vi "UnloadAction.vi"(8 "error in (no error)":errorcluster caption="entrée d'erreur (pas d'erreur)", 11 "Tools In":refnum<class "LeafMagnetometer.lvclass"> caption="DNL_LabVIEW Object in") -> (0 "error out":errorcluster caption="sortie d'erreur", 3 "Tools Out":refnum<class "LeafMagnetometer.lvclass"> caption="DNL_LabVIEW Object out")   [LabVIEW 2019, in "LeafMagnetometer.lvclass"]
uses:
  LeafMagnetometer.lvclass
  C:/Programmes Labview/LabscanV1A/DevicesClass/BaseDevice/BaseDevice.lvclass
  BaseDevice/BaseDevice.lvclass
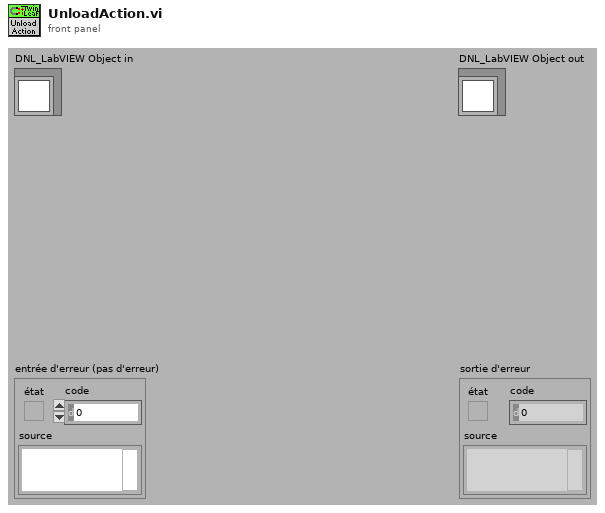
[diagram p1: front panel]
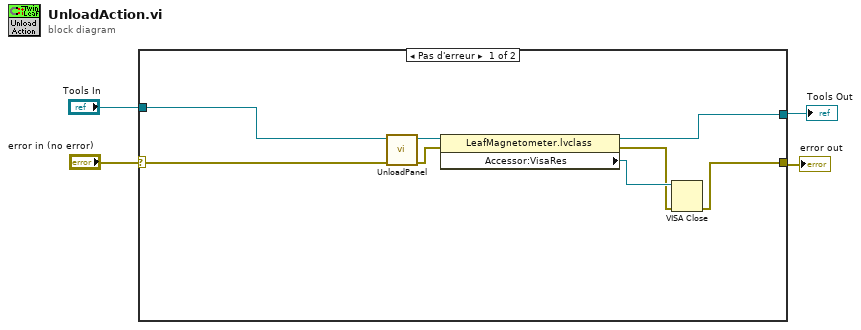
[diagram p0: block diagram]
diagram:
  n1 = case shown="Pas d'erreur" "error in (no error)" {
    selector: "error in (no error)" -> [w11 w13]
    tunnel: [w5 w13] -> w3
    tunnel: [w9 w14] -> w2
    tunnel: "Tools In" -> [w10 w14]
    frame No Error {
      n2 = call "UnloadPanel.vi"("error in (no error)"=w11, "Device en entrée"=w10) -> ("error out"=w7:errorcluster, "Device en sortie"=w12:refnum<class "LeafMagnetometer.lvclass">)  [unwired: 8 in]
      n3 = property class="LeafMagnetometer.lvclass"(reference=w12, error in=w7) -> (reference out=w9:refnum<class "LeafMagnetometer.lvclass">, error out=w6:errorcluster, "Accessor:VisaRes"=w8:refnum<visa-resource-name>)
      n4 = VISA Close(VISA resource name=w8, error in (no error)=w6) -> (error out=w5:errorcluster)
    }
    frame Error {
    }
  }
  "error out" <- w3
  "Tools Out" <- w2
